vi "New Test File Handler.vi"(11 "log directory":path) -> (3 "test file handler":refnum<class "File Handler.lvclass">)   [LabVIEW 2018]
uses:
  api/configuration/handlers/file_handler/File Handler.lvclass
  api/configuration/formatters/format_string_formatter/Format String.lvclass
  C:/Users/Colin/Documents/software_projects/labview/glog/src/api/extension/formatter_interface/Formatter.lvclass
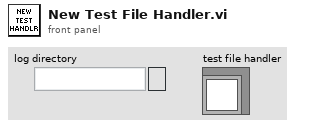
[diagram p1: front panel]
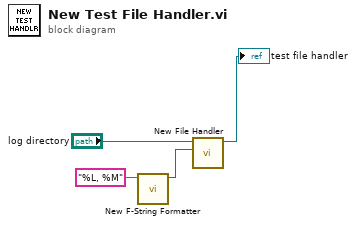
[diagram p0: block diagram]
diagram:
  n1 = call "New F-String Formatter.vi"("format string (\"%T | %L | %M\")"="%L, %M" ("format string (\"%T | %L | %M\")")) -> ("new f-string formatter"=w3:refnum<class "Format String.lvclass">)  [unwired: 10 in]
  n2 = call "New File Handler.vi"("formatter (JSON)"=w3, "log directory (<app dir>/logs)"="log directory") -> ("file handler"=→"test file handler":refnum<class "File Handler.lvclass">)  [unwired: 9 in]
